vi "Laurel Collect Continuous.vi"(7 "stop":bool, 8 "Error In":errorcluster, 10 "Send Command":T1(ring)=enum."Reading: Item 1", 11 "VISA Input":refnum<visa-resource-name>="LaurelLNET") -> (0 "Error Out":errorcluster, 2 "Output":dbl format="%.2f")   [LabVIEW 2016]
uses:
  <vilib>/Instr/_visa.llb/VISA Open Access Mode.ctl
panel:
  out "Previous Value":dbl
  out "Loop Speed":u32
  out "read buffer":string
  in  "Scan Rate":u32=500
  # "Laurel Electronics LNET Continuous Read"
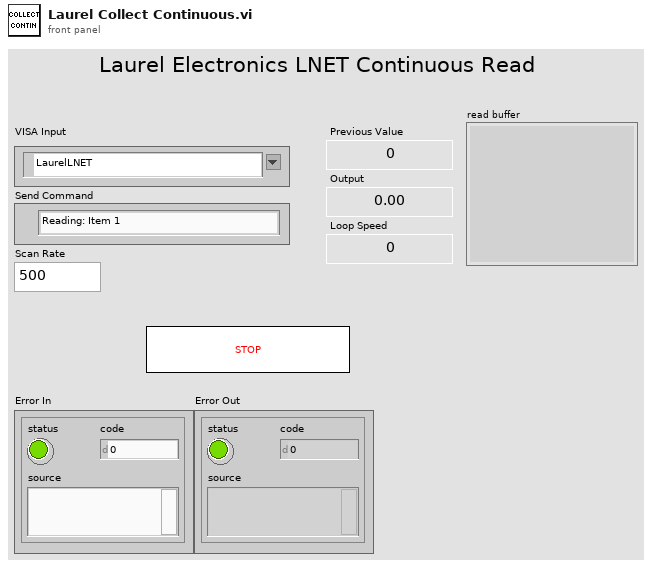
[diagram p1: front panel]
types:
  T1 = enum16{"Command Mode", "Cold Reset", "Function Reset", "Reading: All Active Items", "Reading: Item 1", "Reading: Item 2", "Reading: Item 3"}
  T2 = typedef "VISA Open Access Mode.ctl" = u32
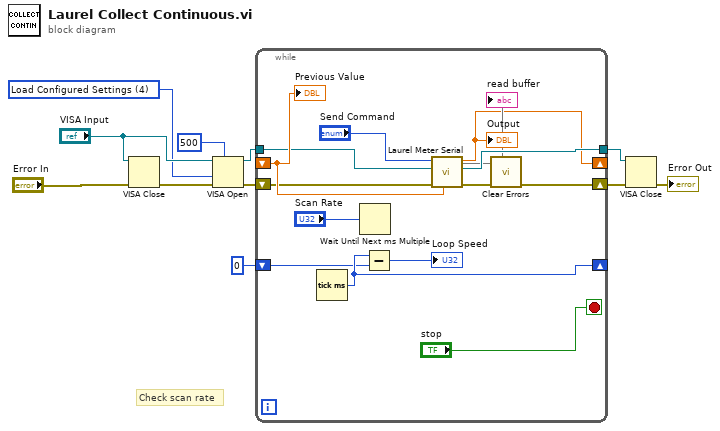
[diagram p0: block diagram]
diagram:
  w3 = T2 4 items=["VISA Defaults"=0, "Exclusive Lock"=1, "Load Configured Settings"=4] ("Access Mode")
  # "Check scan rate"
  n1 = VISA Close(VISA resource name="VISA Input", error in (no error)="Error In") -> (error out=w6:errorcluster)
  n2 = VISA Open(timeout (0)=u32 500 ("VISA Open timeout (0)"), access mode=w3, error in (no error)=w6, VISA resource name="VISA Input") -> (VISA resource name=w8:refnum<visa-resource-name>, error out=w7:errorcluster)  [unwired: 1 in]
  n3 = while {
    shift-right: [w14] -> w9
    shift-left: w7 -> [w12]
    shift-right: [w21] -> _
    shift-left: u32 0 -> [w20]
    tunnel: [w19] -> w10
    tunnel: w8 -> [w13]
    shift-right: [w17] -> _
    shift-left: _ -> [w16]
    stop <- "stop" stop-if-true
    n4 = Tick Count (ms)() -> (millisecond timer value=w21:u32)
    n5 = Wait Until Next ms Multiple(millisecond multiple="Scan Rate") -> ()  [unwired: 1 out]
    n6 = Subtract(x=w21, y=w20) -> (x-y=→"Loop Speed":u32)
    n7 = call "Laurel Meter Serial.vi"(6:w16, "error in (no error)"=w12, "VISA Input"=w13, "Laurel Serial Commands"="Send Command") -> ("error out"=w15:errorcluster, "VISA Output"=w19:refnum<visa-resource-name>, "Output"=w17:dbl, 5:→"read buffer")  [unwired: 4 in]
    "Output" <- w17
    n8 = call <vilib>:"Clear Errors.vi"("error in (no error)"=w15) -> ("error out"=w14:errorcluster)  [unwired: 5 in, 1 out]
    "Previous Value" <- w16
  }
  n9 = VISA Close(VISA resource name=w10, error in (no error)=w9) -> (error out=→"Error Out":errorcluster)
